vi "indexSectionForEntry.vi"(8 "rowNum":i32, 11 "tbl":string[][](array[string])) -> (0 "rowNumAtWhichSecExist":i32, 3 "indexSection":string)   [LabVIEW 2010]
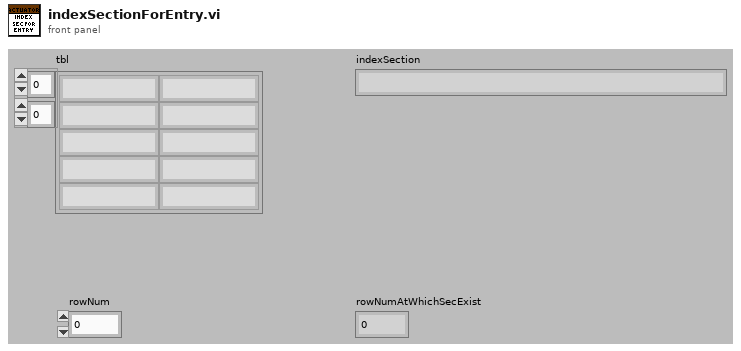
[diagram p1: front panel]
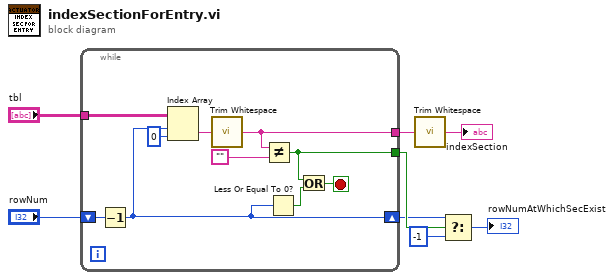
[diagram p0: block diagram]
diagram:
  n1 = while {
    shift-right: [w10] -> w3
    shift-left: "rowNum" -> [w14]
    tunnel: "tbl" -> [w18]
    tunnel: [w11] -> w6
    tunnel: [w9] -> w4
    stop <- w12 stop-if-true
    n2 = Decrement(x=w14) -> (x-1=w10:i32)
    n3 = Index Array(array=w18, index (row)=w10, index (col)=0 ("disabled index (col)")) -> (element=w16:string)
    n4 = call <vilib>:"Trim Whitespace.vi"("string"=w16) -> ("trimmed string"=w11:string)  [unwired: 1 in]
    n5 = Not Equal?(x=w11, y="") -> (x != y?=w9:bool)
    n6 = Less Or Equal To 0?(x=w10) -> (x <= 0?=w13:bool)
    n7 = Or(x=w9, y=w13) -> (x .or. y?=w12:bool)
  }
  n8 = call <vilib>:"Trim Whitespace.vi"("string"=w6) -> ("trimmed string"=→"indexSection":string)  [unwired: 1 in]
  n9 = Select(t=w3, s=w4, f=-1) -> (s? t:f=→"rowNumAtWhichSecExist":i32)
